vi "GetLastParent.vi"(0 "Parent Ref In":refnum<vi>[](array[refnum])) -> (4 "Last Parent Ref":refnum<vi>)   [LabVIEW 2019, in "JsonToCluster.lvlib"]
doc: "This VI gets last parent reference in the reference array"
uses:
  JsonToCluster.lvlib
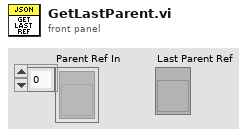
[diagram p1: front panel]
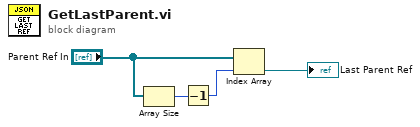
[diagram p0: block diagram]
diagram:
  n1 = Array Size(array="Parent Ref In") -> (size(s)=w1:i32)
  n2 = Decrement(x=w1) -> (x-1=w3:i32)
  n3 = Index Array(array="Parent Ref In", index=w3) -> (element=→"Last Parent Ref":refnum<vi>)
